vi "ChangeLeftSubpanel.vi"(8 "error in (no error)":errorcluster, 10 "Left Active":i32, 11 "MAUI in":refnum<class "MAUI.lvclass">) -> (0 "error out":errorcluster, 3 "MAUI out":refnum<class "MAUI.lvclass">)   [LabVIEW 2016, in "MAUI.lvclass"]
uses:
  MAUI.lvclass
  <vilib>/Levylab/Embedded SMO UI/EmbeddedSMO.lvclass
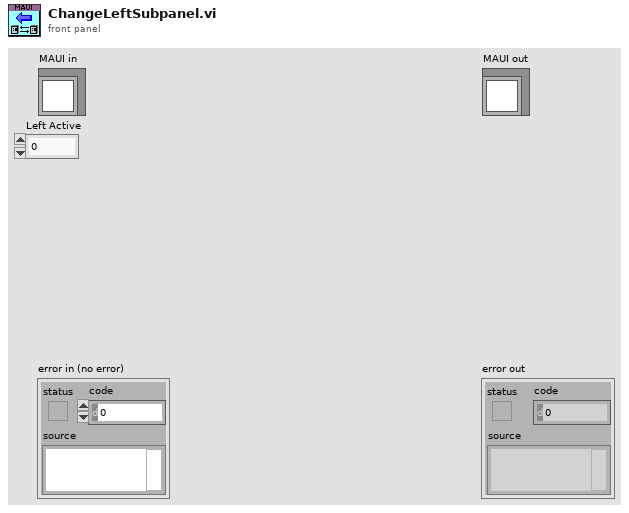
[diagram p1: front panel]
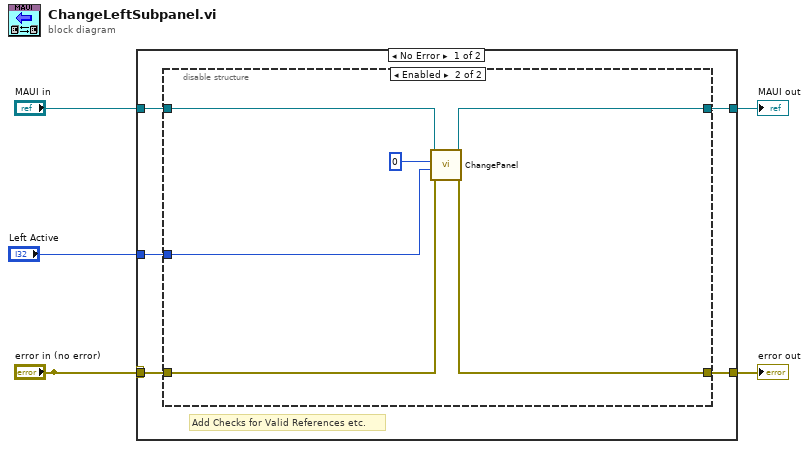
[diagram p0: block diagram]
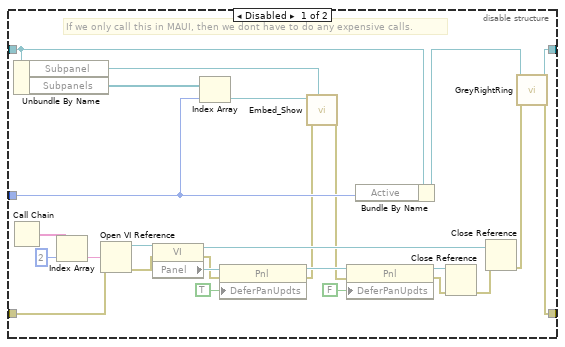
[diagram p2: hidden frame]
diagram:
  n1 = case shown="No Error" "error in (no error)" {
    selector: "error in (no error)" -> [_ w44]
    tunnel: [w7 w44] -> w5
    tunnel: [w8 w43] -> w3
    tunnel: "MAUI in" -> [w9 w43]
    tunnel: "Left Active" -> [w10 _]
    tunnel: "error in (no error)" -> [w6 _]
    frame No Error {
      # "Add Checks for Valid References etc."
      n2 = disable-structure shown="Enabled" {
        disable-tunnel: w10 -> [w36 w37]
        disable-tunnel: w9 -> [w34 w42]
        disable-tunnel: [w32 w41] -> w8
        disable-tunnel: [w31 w39] -> w7
        disable-tunnel: w6 -> [w16 w40]
        frame Disabled {
          # "If we only call this in MAUI, then we dont have to do any expensive calls."
          n3 = Call Chain() -> (call chain=w30:string[])
          n4 = Unbundle By Name(w34) -> ("Subpanel"=w14:refnum<vi>, "Subpanels"=w35:refnum<class "EmbeddedSMO.lvclass">[])
          n5 = Index Array(array=w30, index=2) -> (element=w28:string)
          n6 = Open VI Reference(vi path=w28, error in (no error)=w16) -> (vi reference=w27:refnum<vi>, error out=w23:errorcluster)  [unwired: 4 in]
          n7 = property class="VI"(reference=w27, error in=w23) -> (reference out=w22:refnum<vi>, error out=w24:errorcluster, "Panel"=w26:refnum<vi>)
          n8 = Index Array(array=w35, index=w36) -> (element=w13:refnum<class "EmbeddedSMO.lvclass">)
          n9 = property class="Pnl"(reference=w26, error in=w24, "DeferPanUpdts"=TRUE ("Defer Panel Updates")) -> (reference out=w21:refnum<vi>, error out=w12:errorcluster)
          n10 = call <vilib>:"Embed_Show.vi"("Sub Panel"=w14, "error in (no error)"=w12, "EmbeddedSMO in"=w13) -> ("error out"=w11:errorcluster)  [unwired: 7 in, 1 out]
          n11 = property class="Pnl"(reference=w21, error in=w11, "DeferPanUpdts"=FALSE ("Defer Panel Updates")) -> (reference out=w19:refnum<vi>, error out=w18:errorcluster)
          n12 = Bundle By Name(cluster=w34, "Active"=w36) -> (w33:refnum<class "MAUI.lvclass">)
          n13 = Close Reference(reference=w19, error in (no error)=w18) -> (error out=w17:errorcluster)
          n14 = Close Reference(reference=w22, error in (no error)=w17) -> (error out=w15:errorcluster)
          n15 = call "GreyRightRing.vi"("error in (no error)"=w15, "MAUI in"=w33) -> ("error out"=w31:errorcluster, "MAUI out"=w32:refnum<class "MAUI.lvclass">)  [unwired: 8 in]
        }
        frame Enabled {
          n16 = call "ChangePanel.vi"("error in (no error)"=w40, "Embedded"=w37, "Panel"=0, "MAUI in"=w42) -> ("error out"=w39:errorcluster, "MAUI out"=w41:refnum<class "MAUI.lvclass">)  [unwired: 6 in]
        }
      }
    }
    frame Error {
    }
  }
  "error out" <- w5
  "MAUI out" <- w3
